vi "KE6221 -- PDelta Mode Set Num Low Meas tmp.vi"(0 "Resource In":refnum<visa-resource-name>, 1 "Check For SCPI Errors? (T)":bool=TRUE, 7 "Num Low Meas Per Cycle":T1=enum."2", 11 "error in (no error)":errorcluster) -> (4 "Resource Out (dupl)":refnum<visa-resource-name>, 15 "error out":errorcluster)   [LabVIEW 2014, in "Keithley 622x tmp.lvlib"]
uses:
  Keithley 622x tmp.lvlib
  Typedefs/KE6221 -- PDelta Mode Num Low Meas.ctl
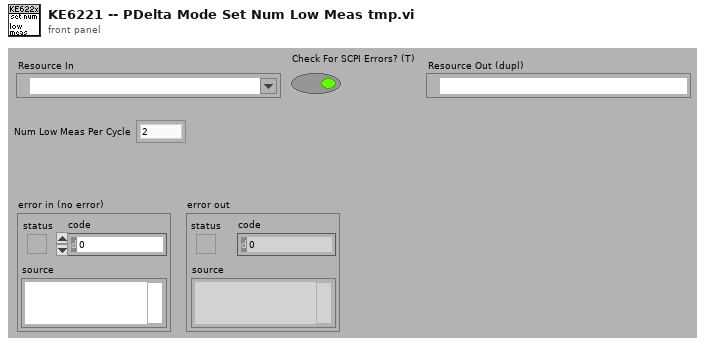
[diagram p1: front panel]
types:
  T1 = typedef "Keithley 622x tmp.lvlib/KE6221 -- PDelta Mode Num Low Meas.ctl" = enum16{"1", "2"}
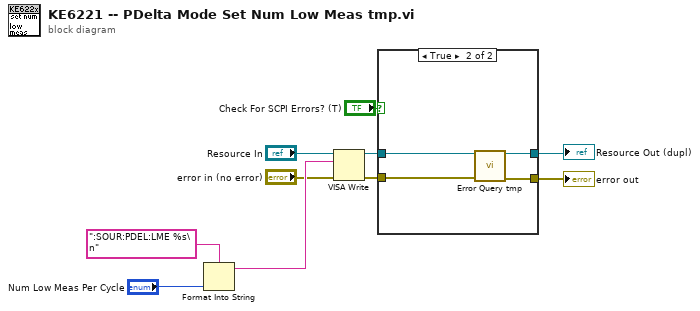
[diagram p0: block diagram]
diagram:
  n1 = Format Into String(format string=":SOUR:PDEL:LME %s\n", "Num Low Meas Per Cycle") -> (resulting string=w8:string)  [unwired: 2 in, 1 out]
  n2 = VISA Write(VISA resource name="Resource In", write buffer=w8, error in (no error)="error in (no error)") -> (VISA resource name out=w5:refnum<visa-resource-name>, error out=w4:errorcluster)  [unwired: 1 out]
  n3 = case shown="True" "Check For SCPI Errors? (T)" {
    tunnel: w5 -> [w12 w16]
    tunnel: w4 -> [w11 w15]
    tunnel: [w11 w14] -> w2
    tunnel: [w12 w13] -> w3
    frame False {
    }
    frame True {
      n4 = call "Error Query tmp.vi"("VISA Resource In"=w16, "error in (no error)"=w15) -> ("VISA Resource Out (dupl)"=w13:refnum<visa-resource-name>, "error out"=w14:errorcluster)  [unwired: 10 in, 2 out]
    }
  }
  "Resource Out (dupl)" <- w3
  "error out" <- w2
